vi "Close File.vi"(8 "error in":errorcluster, 11 "CSV in":refnum<class "CSV.lvclass">) -> (0 "error out":errorcluster, 3 "CSV out":refnum<class "CSV.lvclass">)   [LabVIEW 2017, in "Report_lib.lvlib" / "CSV.lvclass"]
doc: "This method correct closes\n File using File.Refnum"
uses:
  CSV.lvclass
  CSV.lvclass/CSV.ctl
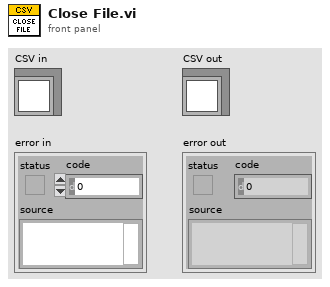
[diagram p1: front panel]
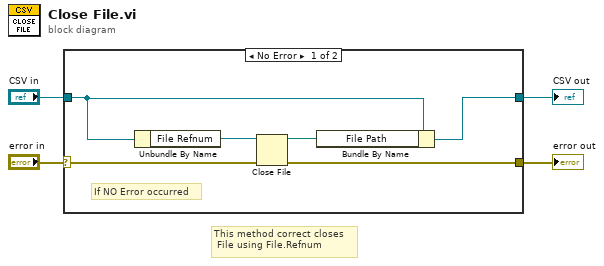
[diagram p0: block diagram]
diagram:
  # "This method correct closes\n File using File.Refnum"
  n1 = case shown="No Error" "error in" {
    selector: "error in" -> [w6 w12]
    tunnel: [w5 w12] -> w3
    tunnel: [w7 w11] -> w1
    tunnel: "CSV in" -> [w8 w11]
    frame No Error {
      # "If NO Error occurred"
      n2 = Unbundle By Name(w8) -> ("File Refnum"=w10:refnum<file>)
      n3 = Close File(refnum=w10, error in=w6) -> (path=w9:path, error out=w5:errorcluster)
      n4 = Bundle By Name(cluster=w8, "File Path"=w9) -> (w7:refnum<class "CSV.lvclass">)
    }
    frame Error {
    }
  }
  "error out" <- w3
  "CSV out" <- w1
